vi "updateStartTrigger.vi"(8 "error in (no error)":errorcluster, 10 "Pane":refnum<vi>, 11 "ICSettingsViewer in":refnum<class "ICSettingsViewer.lvclass">) -> (0 "error out":errorcluster, 2 "Pane out":refnum<vi>, 3 "ICSettingsViewer out":refnum<class "ICSettingsViewer.lvclass">)   [LabVIEW 2011, in "Views.lvlib" / "Camera.lvlib" / "ICSettingsViewer.lvclass"]
uses:
  ICSettingsViewer.lvclass
  ICSettingsViewer.lvclass/ICSettingsViewer.ctl
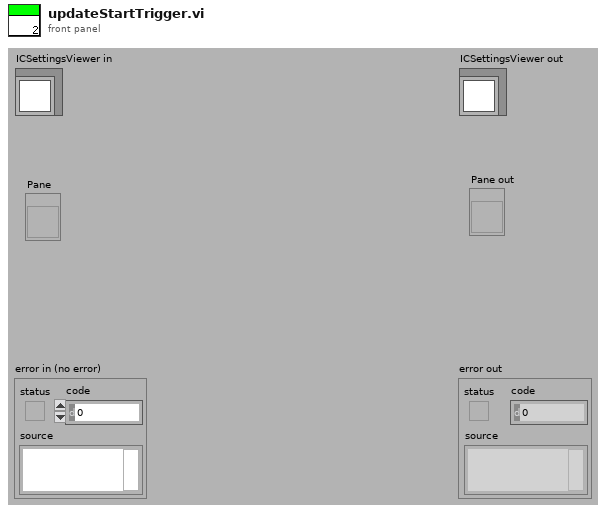
[diagram p1: front panel]
types:
  T1 = enum16{"exposure", "gain", "image_number", "Triggering", "start_trigger"}
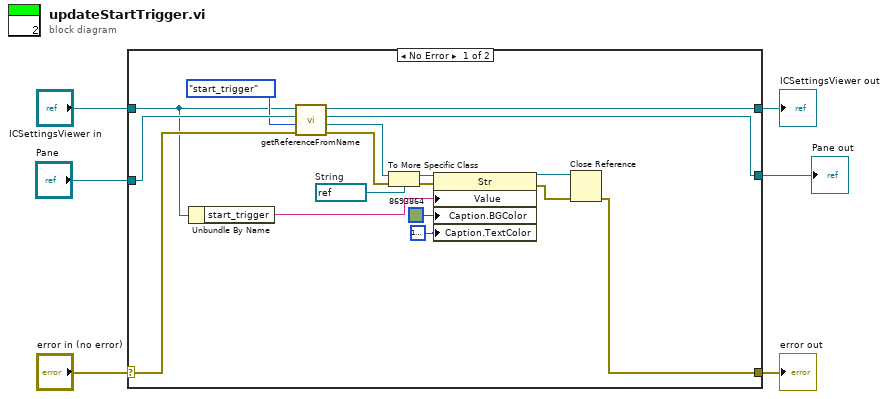
[diagram p0: block diagram]
diagram:
  n1 = case shown="No Error" "error in (no error)" {
    selector: "error in (no error)" -> [w12 w25]
    tunnel: [w11 w25] -> w5
    tunnel: [w8 w24] -> w3
    tunnel: "ICSettingsViewer in" -> [w9 w24]
    tunnel: "Pane" -> [w14 _]
    tunnel: [w7 _] -> w1
    frame No Error {
      w20 = refnum<vi> refnum  # String
      n2 = Unbundle By Name(w9) -> ("start_trigger"=w10:string)
      n3 = call "getReferenceFromName.vi"("error in (no error)"=w12, "referenceName"=T1."start_trigger", "Pane"=w14, "ICSettingsViewer in"=w9) -> ("error out"=w23:errorcluster, "Ctl Refnum"=w19:refnum<vi>, "Pane out"=w7:refnum<vi>, "ICSettingsViewer out"=w8:refnum<class "ICSettingsViewer.lvclass">)  [unwired: 3 in, 1 out]
      n4 = To More Specific Class(target class=w20, reference=w19, error in=w23) -> (specific class reference=w22:refnum<vi>, error out=w21:errorcluster)
      n5 = property class="Str"(reference=w22, error in=w21, "Value"=w10, "Caption.BGColor"=u32 8693864, "Caption.TextColor"=u32 16777222) -> (reference out=w18:refnum<vi>, error out=w17:errorcluster)
      n6 = Close Reference(reference=w18, error in (no error)=w17) -> (error out=w11:errorcluster)
    }
    frame Error {
    }
  }
  "error out" <- w5
  "ICSettingsViewer out" <- w3
  "Pane out" <- w1
